vi "ADC Read Voltage.vi"(4 "Calibration factor":dbl=3.023, 8 "Bit depth":u8 max=3 step=1, 11 "VISA Refnum in":refnum<visa-resource-name>) -> (0 "Voltage in V":dbl, 1 "Configuration byte":u8, 3 "VISA Refnum out":refnum<visa-resource-name>)   [LabVIEW 2015]
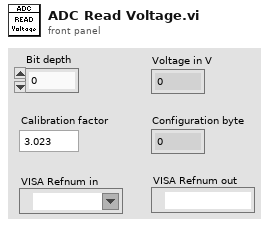
[diagram p1: front panel]
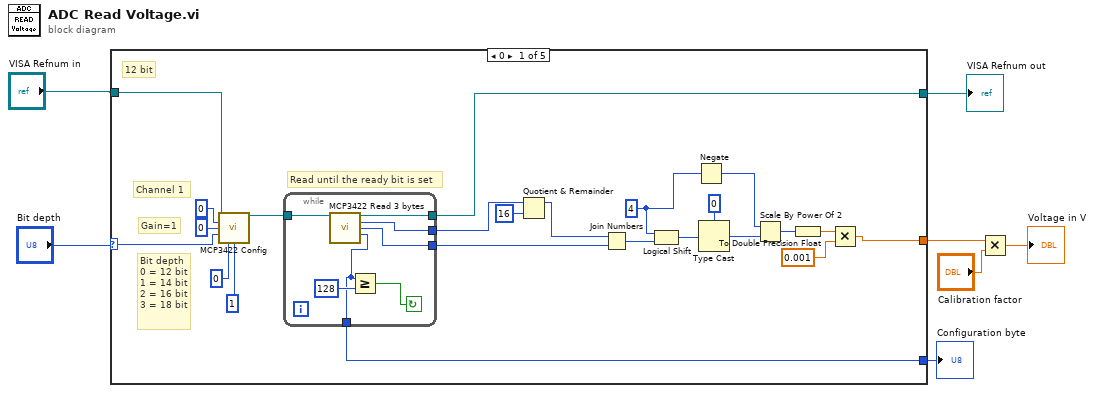
[diagram p0: block diagram]
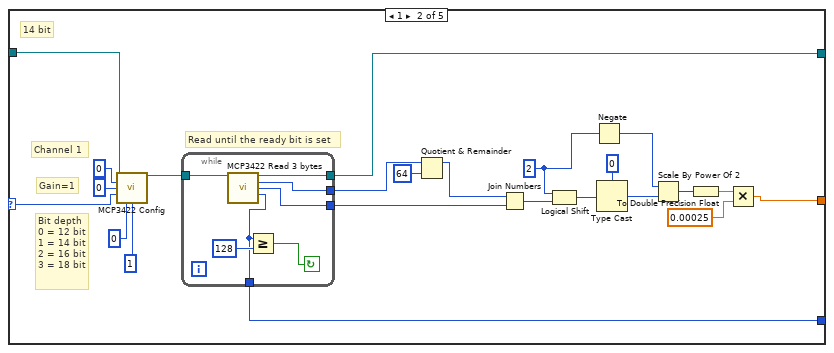
[diagram p2: hidden frame]
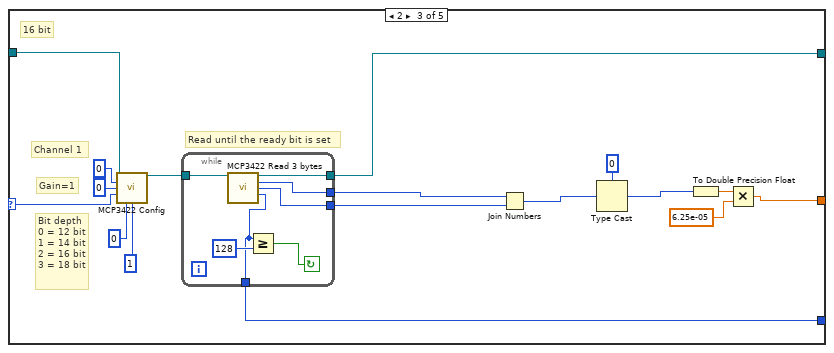
[diagram p3: hidden frame]
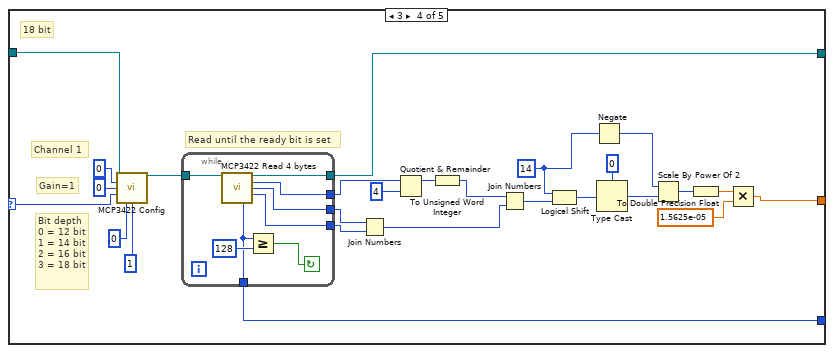
[diagram p4: hidden frame]
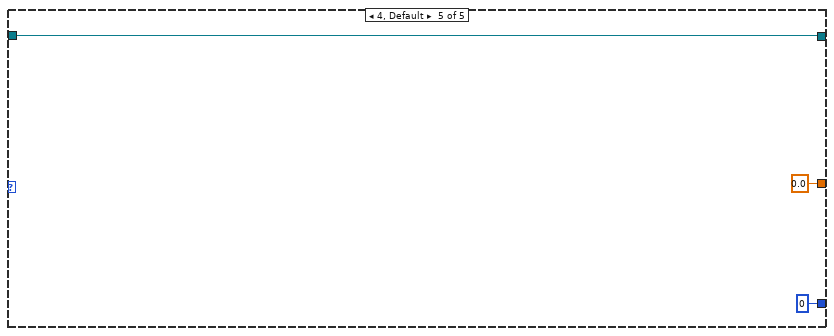
[diagram p5: hidden frame]
diagram:
  n1 = case shown="0" "Bit depth" {
    selector: "Bit depth" -> [w15 w45 w75 w94 _]
    tunnel: "VISA Refnum in" -> [w16 w46 w76 w96 w128]
    tunnel: [w14 w44 w74 w95 w128] -> w6
    tunnel: [w9 w39 w69 w93 0.0] -> w4
    tunnel: [w8 w38 w68 w92 u8 0 ("configuration byte")] -> w1
    frame 0 {
      w20 = i16 4 ("y")
      # "Bit depth\n0 = 12 bit\n1 = 14 bit\n2 = 16 bit\n3 = 18 bit"
      # "12 bit"
      # "Read until the ready bit is set"
      # "Gain=1"
      # "Channel 1"
      n2 = call "MCP3422 Config.vi"("VISA Refnum in"=w16, "Channel selection"=u8 0, "Gain selection"=u8 0, "Sample rate selection"=w15, "Continuous conversion"=u8 0, "Initiate conversion"=u8 1) -> ("VISA Refnum out"=w26:refnum<visa-resource-name>)  [unwired: 8 in, 1 out]
      n3 = while {
        tunnel: w26 -> [w35]
        tunnel: [w34] -> w14
        tunnel: [w33] -> w11
        tunnel: [w32] -> w13
        tunnel: [w31] -> w8
        stop <- w36 continue-if-true
        n4 = call "MCP3422 Read 3 bytes.vi"("VISA Refnum in"=w35) -> ("VISA Refnum out"=w34:refnum<visa-resource-name>, "1st data byte"=w33:u8, "2nd data byte"=w32:u8, "configuration byte"=w31:u8)  [unwired: 10 in, 1 out]
        n5 = Greater Or Equal?(x=w31, y=u8 128) -> (x >= y?=w36:bool)
      }
      n6 = Quotient & Remainder(x=w11, y=u8 16) -> (x-y*floor(x/y)=w12:u8)  [unwired: 1 out]
      n7 = Join Numbers(hi=w12, lo=w13) -> ((hi.lo)=w24:u16)
      n8 = Logical Shift(y=w20, x=w24) -> (x << y=w22:u16)
      n9 = Negate(x=w20) -> (-x=w17:i16)
      n10 = Type Cast(type=i16 0, x=w22) -> (*(type *) &x=w21:i16)
      n11 = Scale By Power Of 2(n=w17, x=w21) -> (x*2^n=w19:i16)
      n12 = To Double Precision Float(number=w19) -> (double precision float=w18:dbl)
      n13 = Multiply(x=w18, y=0.001) -> (x*y=w9:dbl)
    }
    frame 1 {
      w50 = i16 2 ("y")
      # "Bit depth\n0 = 12 bit\n1 = 14 bit\n2 = 16 bit\n3 = 18 bit"
      # "14 bit"
      # "Read until the ready bit is set"
      # "Gain=1"
      # "Channel 1"
      n14 = call "MCP3422 Config.vi"("VISA Refnum in"=w46, "Channel selection"=u8 0, "Gain selection"=u8 0, "Sample rate selection"=w45, "Continuous conversion"=u8 0, "Initiate conversion"=u8 1) -> ("VISA Refnum out"=w56:refnum<visa-resource-name>)  [unwired: 8 in, 1 out]
      n15 = while {
        tunnel: w56 -> [w65]
        tunnel: [w64] -> w44
        tunnel: [w63] -> w41
        tunnel: [w62] -> w43
        tunnel: [w61] -> w38
        stop <- w66 continue-if-true
        n16 = call "MCP3422 Read 3 bytes.vi"("VISA Refnum in"=w65) -> ("VISA Refnum out"=w64:refnum<visa-resource-name>, "1st data byte"=w63:u8, "2nd data byte"=w62:u8, "configuration byte"=w61:u8)  [unwired: 10 in, 1 out]
        n17 = Greater Or Equal?(x=w61, y=u8 128) -> (x >= y?=w66:bool)
      }
      n18 = Quotient & Remainder(x=w41, y=u8 64) -> (x-y*floor(x/y)=w42:u8)  [unwired: 1 out]
      n19 = Join Numbers(hi=w42, lo=w43) -> ((hi.lo)=w54:u16)
      n20 = Logical Shift(y=w50, x=w54) -> (x << y=w52:u16)
      n21 = Negate(x=w50) -> (-x=w47:i16)
      n22 = Type Cast(type=i16 0, x=w52) -> (*(type *) &x=w51:i16)
      n23 = Scale By Power Of 2(n=w47, x=w51) -> (x*2^n=w49:i16)
      n24 = To Double Precision Float(number=w49) -> (double precision float=w48:dbl)
      n25 = Multiply(x=w48, y=0.00025) -> (x*y=w39:dbl)
    }
    frame 2 {
      # "Bit depth\n0 = 12 bit\n1 = 14 bit\n2 = 16 bit\n3 = 18 bit"
      # "16 bit"
      # "Read until the ready bit is set"
      # "Gain=1"
      # "Channel 1"
      n26 = call "MCP3422 Config.vi"("VISA Refnum in"=w76, "Channel selection"=u8 0, "Gain selection"=u8 0, "Sample rate selection"=w75, "Continuous conversion"=u8 0, "Initiate conversion"=u8 1) -> ("VISA Refnum out"=w80:refnum<visa-resource-name>)  [unwired: 8 in, 1 out]
      n27 = while {
        tunnel: w80 -> [w89]
        tunnel: [w88] -> w74
        tunnel: [w87] -> w72
        tunnel: [w86] -> w73
        tunnel: [w85] -> w68
        stop <- w90 continue-if-true
        n28 = call "MCP3422 Read 3 bytes.vi"("VISA Refnum in"=w89) -> ("VISA Refnum out"=w88:refnum<visa-resource-name>, "1st data byte"=w87:u8, "2nd data byte"=w86:u8, "configuration byte"=w85:u8)  [unwired: 10 in, 1 out]
        n29 = Greater Or Equal?(x=w85, y=u8 128) -> (x >= y?=w90:bool)
      }
      n30 = Join Numbers(hi=w72, lo=w73) -> ((hi.lo)=w71:u16)
      n31 = Type Cast(type=i16 0, x=w71) -> (*(type *) &x=w70:i16)
      n32 = To Double Precision Float(number=w70) -> (double precision float=w77:dbl)
      n33 = Multiply(x=w77, y=6.25e-05) -> (x*y=w69:dbl)
    }
    frame 3 {
      w100 = i16 14 ("y")
      # "Bit depth\n0 = 12 bit\n1 = 14 bit\n2 = 16 bit\n3 = 18 bit"
      # "18 bit"
      # "Read until the ready bit is set"
      # "Gain=1"
      # "Channel 1"
      n34 = call "MCP3422 Config.vi"("VISA Refnum in"=w96, "Channel selection"=u8 0, "Gain selection"=u8 0, "Sample rate selection"=w94, "Continuous conversion"=u8 0, "Initiate conversion"=u8 1) -> ("VISA Refnum out"=w113:refnum<visa-resource-name>)  [unwired: 8 in, 1 out]
      n35 = while {
        tunnel: w113 -> [w123]
        tunnel: [w122] -> w95
        tunnel: [w121] -> w110
        tunnel: [w120] -> w112
        tunnel: [w119] -> w111
        tunnel: [w118] -> w92
        stop <- w124 continue-if-true
        n36 = call "MCP3422 Read 4 bytes.vi"("VISA Refnum in"=w123) -> ("VISA Refnum out"=w122:refnum<visa-resource-name>, "1st data byte"=w121:u8, "2nd data byte"=w120:u8, "3rd data byte"=w119:u8, "configuration byte"=w118:u8)  [unwired: 9 in, 1 out]
        n37 = Greater Or Equal?(x=w118, y=u8 128) -> (x >= y?=w124:bool)
      }
      n38 = Join Numbers(hi=w112, lo=w111) -> ((hi.lo)=w107:u16)
      n39 = Quotient & Remainder(x=w110, y=u8 4) -> (x-y*floor(x/y)=w108:u8)  [unwired: 1 out]
      n40 = To Unsigned Word Integer(number=w108) -> (unsigned 16bit integer=w106:u16)
      n41 = Join Numbers(hi=w106, lo=w107) -> ((hi.lo)=w104:u32)
      n42 = Logical Shift(y=w100, x=w104) -> (x << y=w102:u32)
      n43 = Negate(x=w100) -> (-x=w97:i16)
      n44 = Type Cast(type=0, x=w102) -> (*(type *) &x=w101:i32)
      n45 = Scale By Power Of 2(n=w97, x=w101) -> (x*2^n=w99:i32)
      n46 = To Double Precision Float(number=w99) -> (double precision float=w98:dbl)
      n47 = Multiply(x=w98, y=1.5625e-05) -> (x*y=w93:dbl)
    }
    frame 4, Default {
    }
  }
  "VISA Refnum out" <- w6
  "Configuration byte" <- w1
  n48 = Multiply(x=w4, y="Calibration factor") -> (x*y=→"Voltage in V":dbl)
